vi "Label Targets2.vi"(8 "Score Threshold":dbl=75.0, 9 "Annotate":bool=TRUE, 10 "Targets":T2(array[cluster]) {"Carpet" format="%#_3g"; "Short Aspect" format="%#_3g"; "Trapezoid" format="%#_3g"; "Long Aspect" format="%#_3g"; "Area to CH" format="%#_3g"; "X Mask" format="%#_3g"; "Y Mask" format="%#_3g"}, 11 "Image in":T1) -> (3 "Image out":T1)   [LabVIEW 2014]
doc: "Draw text scores near or on the particle. Scores above the threshold are green and underlined."
uses:
  <vilib>/vision/Image Controls.llb/IMAQ Image.ctl
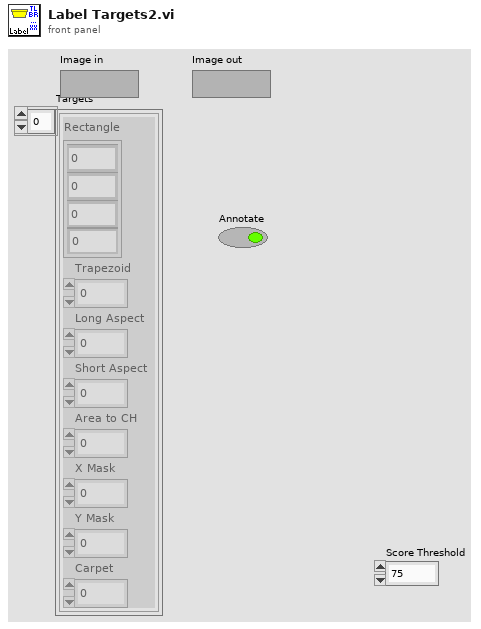
[diagram p1: front panel]
types:
  T1 = typedef "IMAQ Image.ctl" = refnum<image>
  T2 = cluster{"Rectangle":cluster{"Numeric":dbl, "Numeric 2":dbl, "Numeric 3":dbl, "Numeric 5":dbl}, "Trapezoid":dbl, "Long Aspect":dbl, "Short Aspect":dbl, "Area to CH":dbl, "X Mask":dbl, "Y Mask":dbl, "Carpet":dbl}[]
  T3 = cluster{"Desired Font (Application)":enum16{"User-specified Font", "Application Font", "System Font", "Dialog Font"}, "[User-specified Font]":cluster{"Font Name":string, "Size":i16, "Strikeout?":bool, "Italic?":bool, "Underline?":bool, "Outline?":bool, "Shadow?":bool, "Bold?":bool, "Rotation Angle":dbl}, "Horizontal Alignment":i16, "Vertical Alignment":i16}
  T4 = cluster{"Numeric":dbl, "Numeric 2":dbl, "Numeric 3":dbl, "Numeric 5":dbl}
  T5 = cluster{"Trapezoid":dbl, "Long Aspect":dbl, "Short Aspect":dbl, "Area to CH":dbl, "X Mask":dbl, "Y Mask":dbl, "Carpet":dbl}
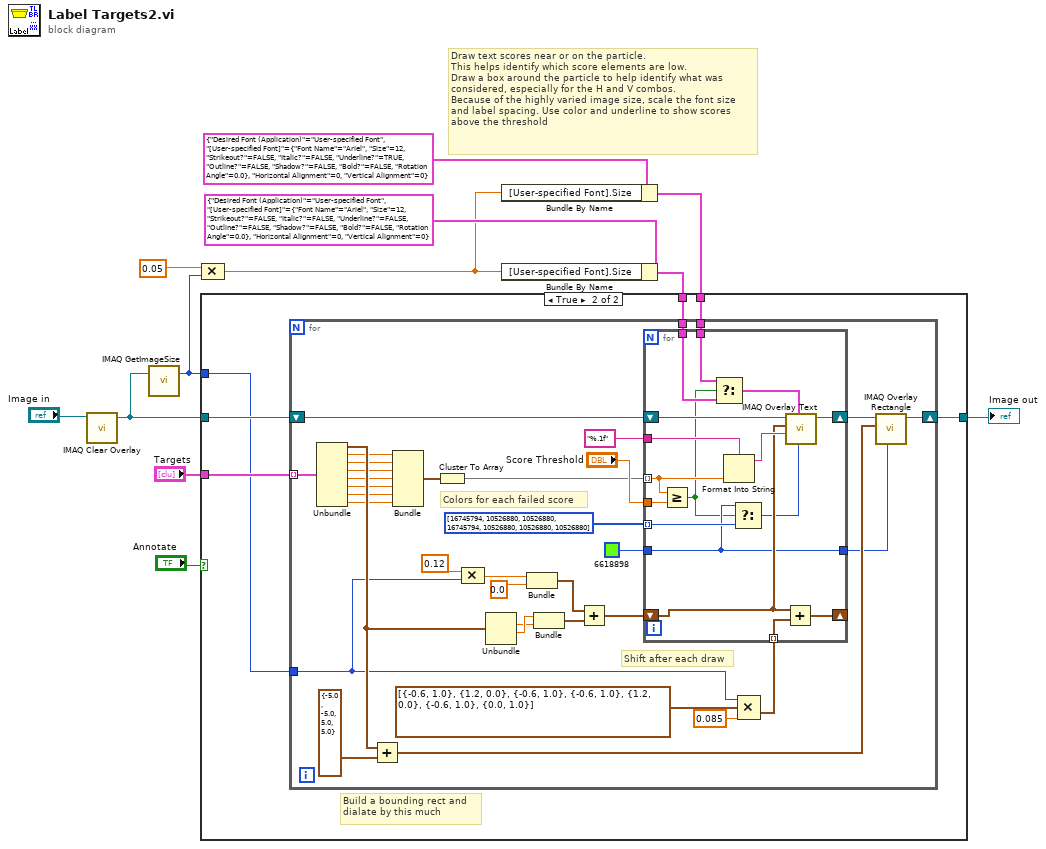
[diagram p0: block diagram]
diagram:
  # "Draw text scores near or on the particle.\nThis helps identify which score elements are low.\nDraw a box around the particle to help identify what was\nconsidered, especially for the H and V combos.\nBecause of the highly varied image size, scale the font size\nand label spacing. Use color and underline to show scores\nabove the threshold"
  n1 = call "IMAQ Clear Overlay"("Image"="Image in") -> ("Image Out"=w4:T1)  [unwired: 2 in, 8 out]
  n2 = call "IMAQ GetImageSize"("Image"=w4) -> ("Y Resolution"=w3:i32)  [unwired: 3 in, 2 out]
  n3 = Compound Arithmetic op=MULTIPLY(0.05, w3) -> (w2:dbl)
  n4 = Bundle By Name(cluster=T3 {"Desired Font (Application)"=enum."User-specified Font", "[User-specified Font]"={"Font Name"="Ariel", "Size"=12, "Strikeout?"=FALSE, "Italic?"=FALSE, "Underline?"=TRUE, "Outline?"=FALSE, "Shadow?"=FALSE, "Bold?"=FALSE, "Rotation Angle"=0.0}, "Horizontal Alignment"=0, "Vertical Alignment"=0} ("Font, Size & Style"), "[User-specified Font].Size"=w2) -> (w5:T3)
  n5 = Bundle By Name(cluster=T3 {"Desired Font (Application)"=enum."User-specified Font", "[User-specified Font]"={"Font Name"="Ariel", "Size"=12, "Strikeout?"=FALSE, "Italic?"=FALSE, "Underline?"=FALSE, "Outline?"=FALSE, "Shadow?"=FALSE, "Bold?"=FALSE, "Rotation Angle"=0.0}, "Horizontal Alignment"=0, "Vertical Alignment"=0} ("Font, Size & Style"), "[User-specified Font].Size"=w2) -> (w6:T3)
  n6 = case shown="True" "Annotate" {
    tunnel: [w13 w19] -> w12
    tunnel: "Targets" -> [_ w18]
    tunnel: w4 -> [w13 w17]
    tunnel: w5 -> [_ w16]
    tunnel: w6 -> [_ w15]
    tunnel: w3 -> [_ w14]
    frame False {
    }
    frame True {
      # "Build a bounding rect and\ndialate by this much"
      n7 = for {
        tunnel: w18 -> [w48] mode=indexing
        shift-right: [w49] -> w19
        shift-left: w17 -> [w54]
        tunnel: w14 -> [w21]
        tunnel: w16 -> [w26]
        tunnel: w15 -> [w25]
        # "Colors for each failed score"
        # "Shift after each draw"
        n8 = Unbundle(w48) -> ("Rectangle"=w42:T4, "Trapezoid"=w40:dbl, "Long Aspect"=w39:dbl, "Short Aspect"=w34:dbl, "Area to CH"=w38:dbl, "X Mask"=w37:dbl, "Y Mask"=w36:dbl, "Carpet"=w35:dbl)
        n9 = Add(x=w42, y=cluster{dbl, dbl, dbl, dbl} {-5.0, -5.0, 5.0, 5.0} ("output cluster")) -> (x+y=w44:cluster{dbl, dbl, dbl, dbl})
        n10 = Bundle("Trapezoid"=w40, "Long Aspect"=w39, "Short Aspect"=w34, "Area to CH"=w38, "X Mask"=w37, "Y Mask"=w36, "Carpet"=w35) -> (w51:T5)  [unwired: 1 in]
        n11 = Cluster To Array(cluster=w51) -> (array=w41:dbl[])
        n12 = Compound Arithmetic op=MULTIPLY(0.12, w21) -> (w22:dbl)
        n13 = Unbundle(w42) -> ("Numeric 2"=w46:dbl, "Numeric 3"=w47:dbl)  [unwired: 2 out]
        n14 = Bundle(w22, 0.0) -> (w24:cluster{dbl, dbl})  [unwired: 1 in]
        n15 = Bundle("Numeric 3"=w47, "Numeric 2"=w46) -> (w45:cluster{"Numeric 3":dbl, "Numeric 2":dbl})  [unwired: 1 in]
        n16 = Add(x=w24, y=w45) -> (x+y=w53:cluster{dbl, dbl})
        n17 = Compound Arithmetic op=MULTIPLY(w21, cluster{dbl, dbl}[] [{-0.6, 1.0}, {1.2, 0.0}, {-0.6, 1.0}, {-0.6, 1.0}, {1.2, 0.0}, {-0.6, 1.0}, {0.0, 1.0}], 0.085) -> (w30:cluster{dbl, dbl}[])
        n18 = for {
          tunnel: w41 -> [w64] mode=indexing
          shift-right: [w67] -> _
          shift-left: w53 -> [w66]
          shift-right: [w68] -> w50
          shift-left: w54 -> [w69]
          tunnel: u32[] [16745794, 10526880, 10526880, 16745794, 10526880, 10526880, 10526880] -> [w65] mode=indexing
          tunnel: "Score Threshold" -> [w63]
          tunnel: w30 -> [w61] mode=indexing
          tunnel: "%.1f" ("format string") -> [w60]
          tunnel: u32 6618898 ("Color") -> [w59]
          tunnel: [w59] -> w32
          tunnel: w26 -> [w58]
          tunnel: w25 -> [w57]
          n19 = Greater Or Equal?(x=w64, y=w63) -> (x >= y?=w56:bool)
          n20 = Select(t=w58, s=w56, f=w57) -> (s? t:f=w55:T3)
          n21 = Format Into String(format string=w60, w64) -> (resulting string=w70:string)  [unwired: 2 in, 1 out]
          n22 = Select(t=w59, s=w56, f=w65) -> (s? t:f=w62:u32)
          n23 = Add(x=w61, y=w66) -> (x+y=w67:cluster{dbl, dbl})
          n24 = call "IMAQ Overlay Text"("Text Color (black)"=w62, "Font, Size & Style"=w55, "String"=w70, "Origin"=w66, "Image"=w69) -> ("Image Out"=w68:T1)  [unwired: 5 in, 1 out]
        }
        n25 = call "IMAQ Overlay Rectangle"("Color"=w32, "Rectangle"=w44, "Image"=w50) -> ("Image Out"=w49:T1)  [unwired: 7 in, 1 out]
      }
    }
  }
  "Image out" <- w12
